vi "Error Module.vi"(7 "command (handle errors)":T1=enum."Handle Errors", 8 "error in":errorcluster, 9 "dynamic event queue reference":T2, 10 "User Interface Control Reference":refnum<queue>, 11 "User Event Control Reference":refnum<queue>) -> (0 "error out":errorcluster, 2 "status":bool)   [LabVIEW 2011]
doc: "Controls access to the Cue data."
uses:
  Controls/Dynamic Event Queue Reference.ctl
  Controls/User Event Control.ctl
  Controls/User Event Action.ctl
  Controls/User Interface Control.ctl
  Controls/User Interface Action.ctl
  Error Module Action.ctl
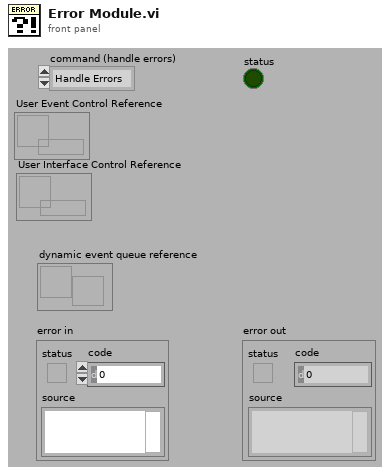
[diagram p1: front panel]
types:
  T1 = typedef "Error Module Action.ctl" = enum16{"Initialize", "Handle Errors", "Report Errors"}
  T2 = typedef "Dynamic Event Queue Reference.ctl" = refnum<user-event>
  T3 = typedef "User Interface Control.ctl" = cluster{"data1":variant, "data2":variant, "action":T4}
  T4 = typedef "User Interface Action.ctl" = enum16{"Initialize", "Update Real Channel", "Update Imag Channel", "Update Re/Im channel @ Hardware Ctrl", "Pulse Sequence", "Visibility Front Panel Controls", "Report Custom Errors", "Set Pulse Sequence Type", "Update Pulse Timings", "Update Transfer Time", "Update Status Bar", "Set Sequence Progress", "Set 90 Degree Pulse Sequence Params", "Set CMPG Pulse Sequence Parms", "Set T1 Pulse Sequence Params", "Stop"}
  T5 = typedef "User Event Control.ctl" = cluster{"data":variant, "action":T6}
  T6 = typedef "User Event Action.ctl" = enum16{"Initialize", "Shutdown", "Start NMR DAQ", "Start NMR DAQ Loop", "Set DDS", "Reset DDS", "Send Pulse", "Set TX SW", "Set RX SW", "Set CutOff Freq1", "Set CutOff Freq2", "Set Gain1", "Set Gain2", "Start AQS", "Configure Device Settings"}
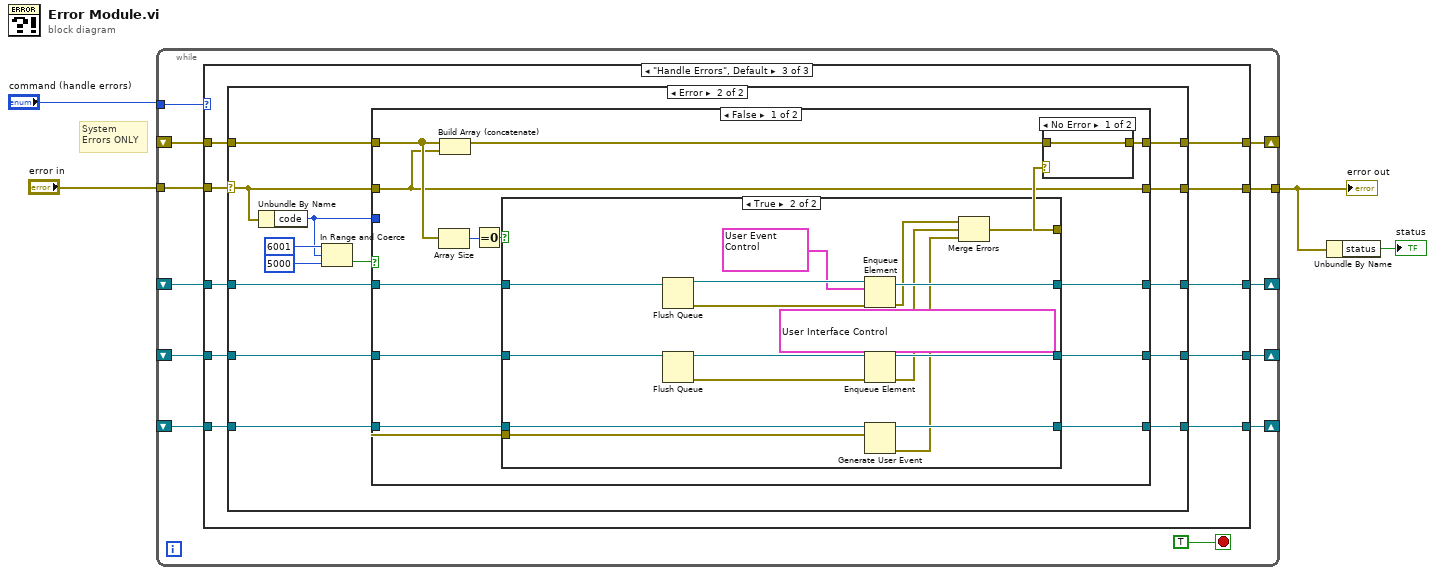
[diagram p0: block diagram]
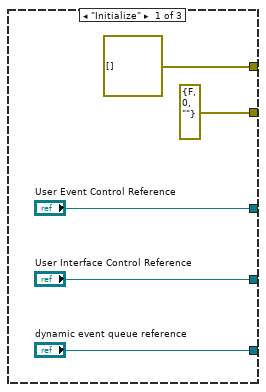
[diagram p2: hidden frame]
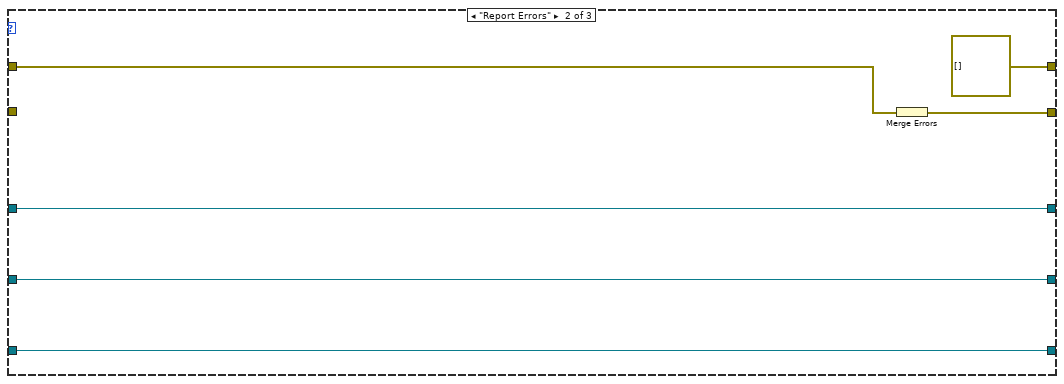
[diagram p3: hidden frame]
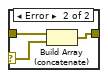
[diagram p5: hidden frame]
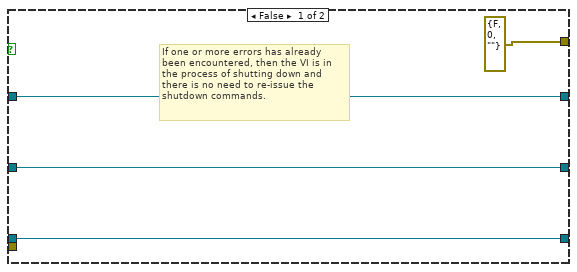
[diagram p6: hidden frame]
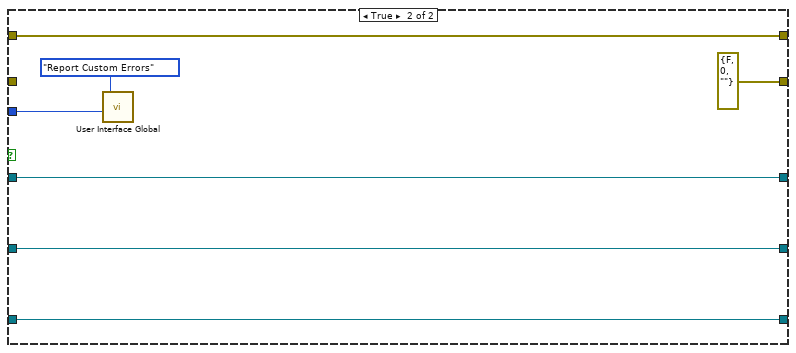
[diagram p7: hidden frame]
diagram:
  # "System\nErrors ONLY"
  n1 = while {
    shift-right: [w12] -> _
    shift-left: _ -> [w14]
    tunnel: "error in" -> [w15]
    tunnel: "command (handle errors)" -> [w13]
    tunnel: [w11] -> w3
    shift-right: [w5] -> _
    shift-left: _ -> [w10]
    shift-right: [w6] -> _
    shift-left: _ -> [w9]
    shift-right: [w7] -> _
    shift-left: _ -> [w8]
    stop <- TRUE stop-if-true
    n2 = case shown="\"Handle Errors\", Default" w13 {
      tunnel: w15 -> [_ _ w37]
      tunnel: [errorcluster[] [] errorcluster[] [] w35] -> w12
      tunnel: w14 -> [_ w26 w36]
      tunnel: [errorcluster {"status"=FALSE, "code"=0, "source"=""} ("error out") w27 w28] -> w11
      tunnel: w10 -> [_ w25 w34]
      tunnel: w9 -> [_ w24 w33]
      tunnel: w8 -> [_ w23 w32]
      tunnel: ["dynamic event queue reference" w23 w29] -> w7
      tunnel: ["User Interface Control Reference" w24 w30] -> w6
      tunnel: ["User Event Control Reference" w25 w31] -> w5
      frame "Initialize" {
      }
      frame "Report Errors" {
        n3 = Merge Errors(w26) -> (w27:errorcluster)
      }
      frame "Handle Errors", Default {
        n4 = case shown="Error" w37 {
          selector: w37 -> [w38 w48]
          tunnel: [w42 w55] -> w35
          tunnel: w36 -> [w42 w56]
          tunnel: w34 -> [w41 w54]
          tunnel: w33 -> [w40 w53]
          tunnel: w32 -> [w39 w52]
          tunnel: [w39 w51] -> w29
          tunnel: [w40 w50] -> w30
          tunnel: [w41 w49] -> w31
          tunnel: [w38 w43] -> w28
          frame No Error {
          }
          frame Error {
            n5 = Unbundle By Name(w48) -> ("code"=w44:i32)
            n6 = In Range and Coerce(upper limit=6001, x=w44, lower limit=5000) -> (In Range?=w45:bool)  [unwired: 1 out]
            n7 = case shown="False" w45 {
              tunnel: w56 -> [w69 w101]
              tunnel: [w65 w101] -> w55
              tunnel: w54 -> [w63 w100]
              tunnel: w53 -> [w62 w99]
              tunnel: w52 -> [w61 w98]
              tunnel: [w60 w98] -> w51
              tunnel: [w59 w99] -> w50
              tunnel: [w58 w100] -> w49
              tunnel: w48 -> [w57 _]
              tunnel: w44 -> [_ w95]
              tunnel: [w57 errorcluster {"status"=FALSE, "code"=0, "source"=""} ("error IO")] -> w43
              frame False {
                n8 = Array Size(array=w69) -> (size(s)=w67:i32)
                n9 = Build Array (concatenate)(w69, w57) -> (w66:errorcluster[])
                n10 = Equal To 0?(x=w67) -> (x = 0?=w68:bool)
                n11 = case shown="True" w68 {
                  tunnel: [errorcluster {"status"=FALSE, "code"=0, "source"=""} ("error out") w83] -> w64
                  tunnel: w57 -> [_ w87]
                  tunnel: w63 -> [w76 w94]
                  tunnel: w62 -> [w75 w93]
                  tunnel: w61 -> [w74 w88]
                  tunnel: [w74 w86] -> w60
                  tunnel: [w75 w85] -> w59
                  tunnel: [w76 w84] -> w58
                  frame False {
                    # "If one or more errors has already \nbeen encountered, then the VI is in \nthe process of shutting down and \nthere is no need to re-issue the \nshutdown commands."
                  }
                  frame True {
                    n12 = Flush Queue(queue=w94) -> (queue out=w92:refnum<queue>, error out=w89:errorcluster)  [unwired: 1 in, 1 out]
                    n13 = Flush Queue(queue=w93) -> (queue out=w91:refnum<queue>, error out=w90:errorcluster)  [unwired: 1 in, 1 out]
                    n14 = Enqueue Element(queue=w92, element=T5 {"data"=variant, "action"=enum."Shutdown"}, error in (no error)=w89) -> (queue out=w84:refnum<queue>, error out=w82:errorcluster)  [unwired: 1 in, 1 out]
                    n15 = Enqueue Element(queue=w91, element=T3 {"data1"=variant, "data2"=variant, "action"=enum."Stop"}, error in (no error)=w90) -> (queue out=w85:refnum<queue>, error out=w81:errorcluster)  [unwired: 1 in, 1 out]
                    n16 = Generate User Event(user event=w88, event data cluster=w87) -> (user event out=w86:T2, error out=w80:errorcluster)  [unwired: 1 in]
                    n17 = Merge Errors(w82, w81, w80) -> (w83:errorcluster)
                  }
                }
                n18 = case shown="No Error" w64 {
                  selector: w64 -> [_ w71]
                  tunnel: w66 -> [w70 w73]
                  tunnel: [w70 w72] -> w65
                  frame No Error {
                  }
                  frame Error {
                    n19 = Build Array (concatenate)(w73, w71) -> (w72:errorcluster[])
                  }
                }
              }
              frame True {
                n20 = call "User Interface Global.vi"("data1"=w95, "action"=User_Interface_Action."Report Custom Errors") -> ()  [unwired: 9 in, 1 out]
              }
            }
          }
        }
      }
    }
  }
  "error out" <- w3
  n21 = Unbundle By Name(w3) -> ("status"=→"status":bool)
